vi "Write Linkage Errors.vi"(8 "error in (no error)":errorcluster, 10 "Linkage Errors":errorcluster[](array[cluster]), 11 "Test Runner in":refnum<class "Test Runner.lvclass">) -> (0 "error out":errorcluster, 3 "Test Runner out":refnum<class "Test Runner.lvclass">)   [LabVIEW 2020, in "Caraya.lvlib" / "Test Runner.lvclass"]
doc: "Writes a list of errors from linkage info\n\n(Leave error array empty to clear all errors)"
uses:
  Test Runner.lvclass
  Test Runner.lvclass/Test Runner.ctl
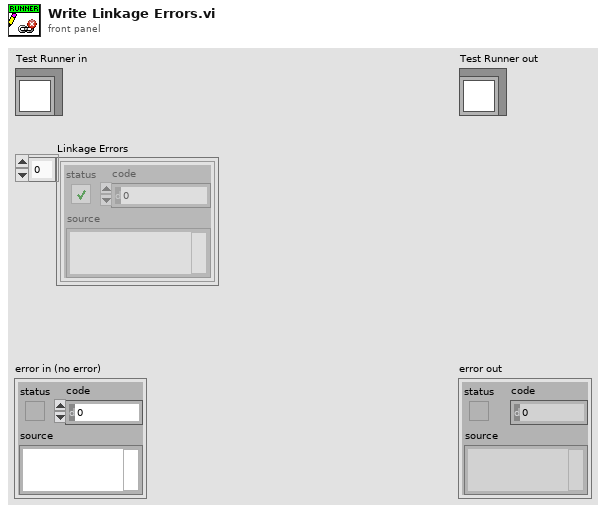
[diagram p1: front panel]
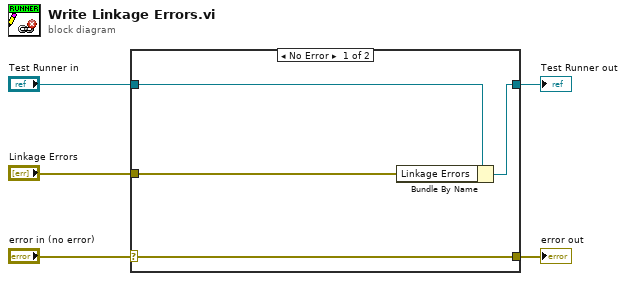
[diagram p0: block diagram]
diagram:
  n1 = case shown="No Error" "error in (no error)" {
    selector: "error in (no error)" -> [w9 w10]
    tunnel: [w9 w10] -> w4
    tunnel: [w7 w11] -> w2
    tunnel: "Test Runner in" -> [w8 w11]
    tunnel: "Linkage Errors" -> [w6 _]
    frame No Error {
      n2 = Bundle By Name(cluster=w8, "Linkage Errors"=w6) -> (w7:refnum<class "Test Runner.lvclass">)
    }
    frame Error {
    }
  }
  "error out" <- w4
  "Test Runner out" <- w2
